vi "Refnum Names.vi"() -> ()   [LabVIEW 2014]
panel:
  in  "DB/Gyro Custom":string="DB/Gyro Gain"
  in  "DB/Gyro Choice":string="DB/Gyro Choice"
  in  "DB/Gyro":string="DB/Gyro"
  in  "Unused":string
  in  "Gyro":string="Gyro"
  in  "DB/Auto Mode":string="DB/Auto Mode"
  in  "DB/Wiggles":string="DB/Wiggles"
  in  "DB/Time":string="DB/Time"
  in  "DB/Drive From Step":string="DB/Drive Forward After Can"
  in  "DB/Right Turn":string="DB/Auto 7 Right"
  in  "DB/Motors":string="RobotDrive Motors"
  in  "CB Sol":string="CBSol"
  in  "Arm Sol":string="Grabber"
  in  "Mast Sol":string="Mast"
  in  "CB Motor":string="CBPWM"
  in  "Arm Motor":string="Arm"
  in  "Drive Motors":string="Drive"
  in  "Gamepad":string="Joystick 1"
  in  "Joystick W/Rotation":string="Joystick 0"
  # "Motors"
  # "Solenoids"
  # "Joysticks"
  # "Dashboard"
  # "Analog"
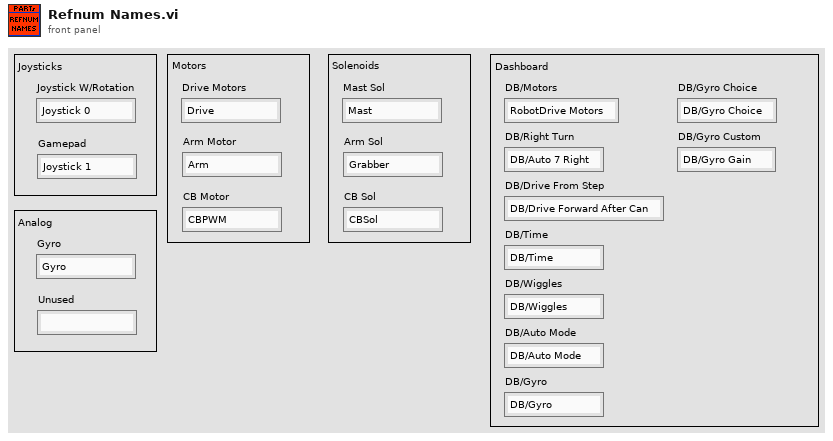
[diagram p1: front panel]
diagram:
